vi "CRYAPI Pic Get FloatSize.vi"(7 "sAction":string, 9 "tFrameTAB":T2, 11 "tFrame":T2) -> (1 "FPPanelBound_Out":T1, 3 "tFrame_Out":T2)   [LabVIEW 2013]
uses:
  <vilib>/Utility/miscctls.llb/LVRectTypeDef.ctl
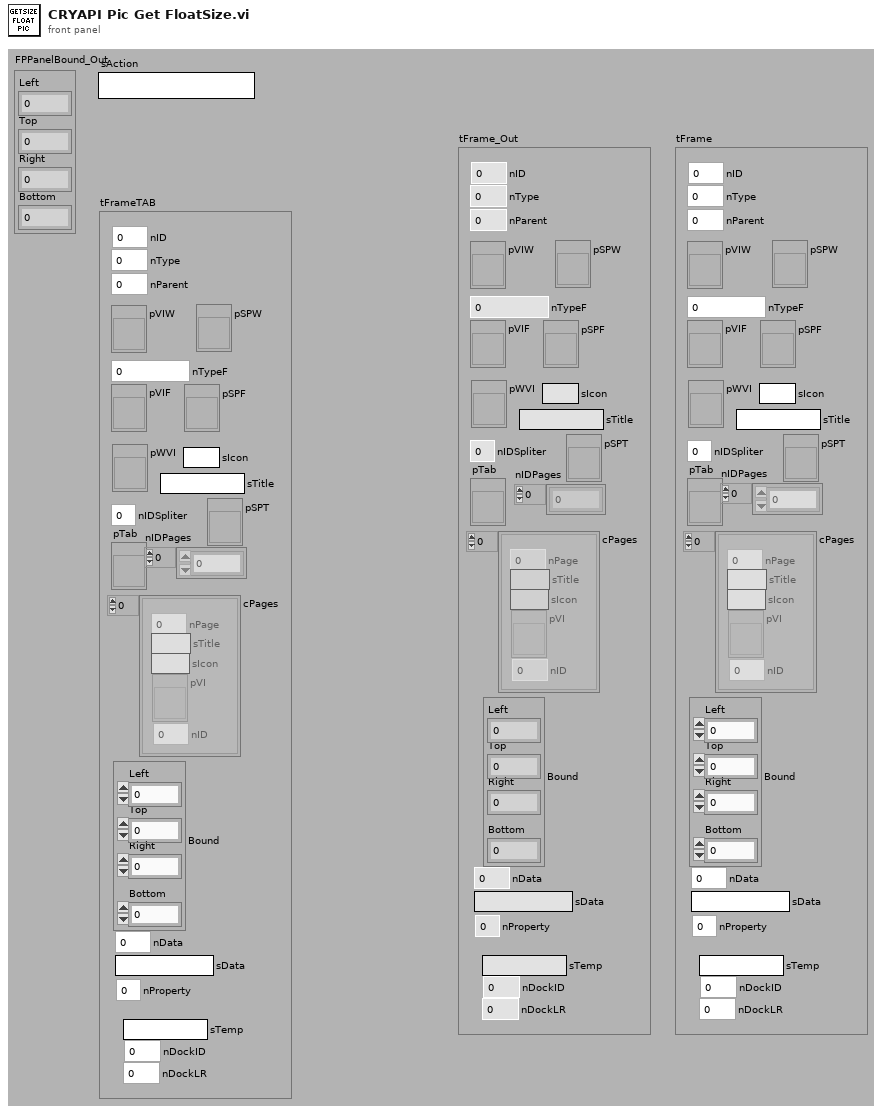
[diagram p1: front panel]
types:
  T1 = typedef "LVRectTypeDef.ctl" = cluster{"Left":i16, "Top":i16, "Right":i16, "Bottom":i16}
  T2 = cluster{"nType":i32, "nParent":i32, "pVIW":refnum<vi>, "pSPW":refnum<vi>, "nTypeF":i32, "pVIF":refnum<vi>, "pSPF":refnum<vi>, "nIDSpliter":i32, "nProperty":i32, "Bound":T1, "nID":i32, "nData":i32, "sData":string, "pWVI":refnum<vi>, "sTitle":string, "cPages":cluster{"nPage":i32, "sTitle":string, "sIcon":string, "pVI":refnum<vi>, "nID":i32}[], "pTab":refnum<vi>, "nIDPages":i32[], "pSPT":refnum<vi>, "sTemp":string, "nDockID":i32, "nDockLR":i32, "sIcon":string}
  T3 = typedef "LVBoundsTypeDef.ctl" = cluster{"Width":u32, "Height":u32}
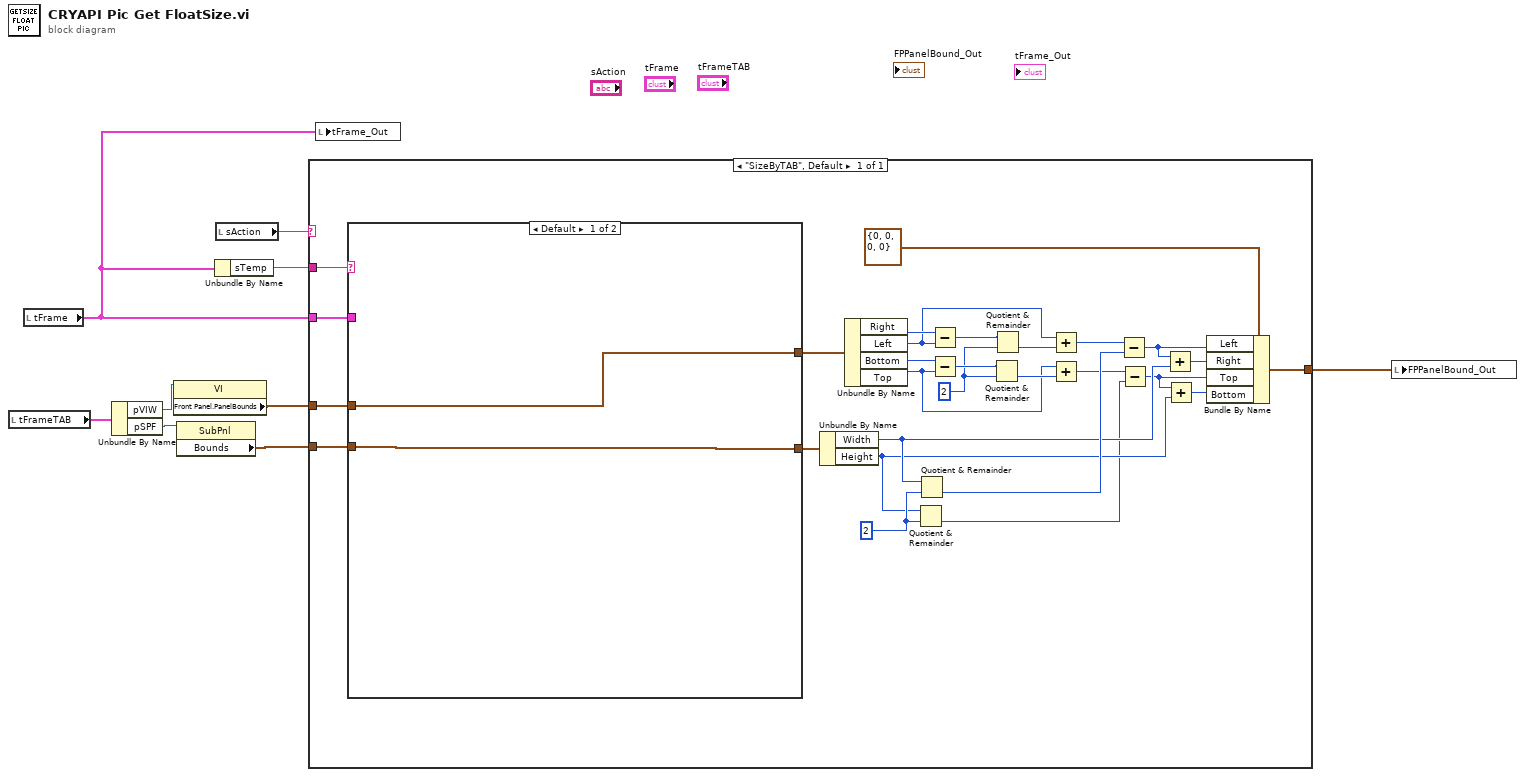
[diagram p0: block diagram]
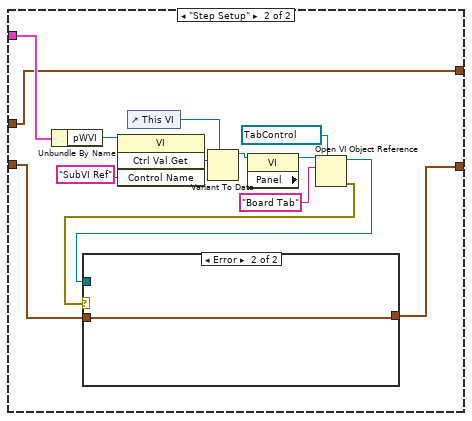
[diagram p2: hidden frame]
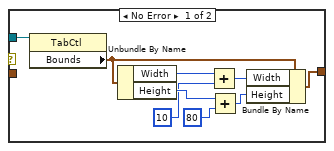
[diagram p3: hidden frame]
diagram:
  n1 = local read "tFrameTAB"() -> (w3:T2)
  n2 = local read "tFrame"() -> (w6:T2)
  n3 = Unbundle By Name(w3) -> ("pVIW"=w4:refnum<vi>, "pSPF"=w5:refnum<vi>)
  n4 = property class="VI"(reference=w4) -> ("Front Panel.PanelBounds"=w2:T1)  [unwired: 1 in, 2 out]
  n5 = property class="SubPnl"(reference=w5) -> ("Bounds"=w1:T3)  [unwired: 1 in, 2 out]
  n6 = Unbundle By Name(w6) -> ("sTemp"=w7:string)
  n7 = local read "sAction"() -> (w8:string)
  n8 = case shown="\"SizeByTAB\", Default" w8 {
    tunnel: [w14] -> w9
    tunnel: w6 -> [w12]
    tunnel: w7 -> [w13]
    tunnel: w2 -> [w11]
    tunnel: w1 -> [w10]
    frame "SizeByTAB", Default {
      w26 = 2
      w30 = 2
      n9 = case shown="Default" w13 {
        tunnel: [w39 w41] -> w37
        tunnel: [w38 w42] -> w27
        tunnel: w12 -> [_ w53]
        tunnel: w11 -> [w39 w41]
        tunnel: w10 -> [w38 w40]
        frame Default {
        }
        frame "Step Setup" {
          n10 = Unbundle By Name(w53) -> ("pWVI"=w52:refnum<vi>)
          n11 = invoke class="VI" method="Ctrl Val.Get"(reference=w52, "Control Name"="SubVI Ref") -> ("Get Control Value Variant"=w50:variant)  [unwired: 2 in, 3 out]
          n12 = control-ref of="This VI"() -> (w49:refnum<vi>)
          n13 = Variant To Data(type=w49, Variant=w50) -> (data=w47:refnum<vi>)  [unwired: 1 in, 1 out]
          n14 = property class="VI" props=["Panel"](reference=w47) -> (reference out=w46:refnum<vi>)  [unwired: 1 in, 2 out]
          n15 = Open VI Object Reference(7:refnum<vi> refnum ("Tab Control"), 10:"Board Tab" ("name/order"), 11:w46) -> (0:w44:errorcluster, 3:w43:refnum<vi>)  [unwired: 1 in]
          n16 = case shown="Error" w44 {
            tunnel: w43 -> [w62 _]
            tunnel: [w56 w63] -> w42
            tunnel: w40 -> [_ w63]
            frame No Error {
              n17 = property class="TabCtl"(reference=w62) -> ("Bounds"=w61:T3)  [unwired: 1 in, 2 out]
              n18 = Unbundle By Name(w61) -> ("Width"=w60:u32, "Height"=w59:u32)
              n19 = Add(x=w60, y=u32 10) -> (x+y=w58:u32)
              n20 = Add(x=w59, y=u32 80) -> (x+y=w57:u32)
              n21 = Bundle By Name(cluster=w61, "Width"=w58, "Height"=w57) -> (w56:T3)
            }
            frame Error {
            }
          }
        }
      }
      n22 = Unbundle By Name(w27) -> ("Width"=w22:u32, "Height"=w16:u32)
      n23 = Unbundle By Name(w37) -> ("Right"=w36:i16, "Left"=w34:i16, "Bottom"=w35:i16, "Top"=w28:i16)
      n24 = Quotient & Remainder(x=w16, y=w26) -> (floor(x/y)=w15:u32)  [unwired: 1 out]
      n25 = Quotient & Remainder(x=w22, y=w26) -> (floor(x/y)=w23:u32)  [unwired: 1 out]
      n26 = Subtract(x=w36, y=w34) -> (x-y=w33:i16)
      n27 = Subtract(x=w35, y=w28) -> (x-y=w31:i16)
      n28 = Quotient & Remainder(x=w31, y=w30) -> (floor(x/y)=w29:i32)  [unwired: 1 out]
      n29 = Quotient & Remainder(x=w33, y=w30) -> (floor(x/y)=w32:i32)  [unwired: 1 out]
      n30 = Add(x=w34, y=w32) -> (x+y=w24:i32)
      n31 = Add(x=w28, y=w29) -> (x+y=w18:i32)
      n32 = Subtract(x=w24, y=w23) -> (x-y=w21:u32)
      n33 = Subtract(x=w18, y=w15) -> (x-y=w17:u32)
      n34 = Add(x=w21, y=w22) -> (x+y=w20:u32)
      n35 = Add(x=w17, y=w16) -> (x+y=w19:u32)
      n36 = Bundle By Name(cluster=T1 {"Left"=0, "Top"=0, "Right"=0, "Bottom"=0} ("Front Panel Window:Panel Bounds"), "Left"=w21, "Right"=w20, "Top"=w17, "Bottom"=w19) -> (w14:T1)
    }
  }
  n37 = local write "tFrame_Out"(w6) -> ()
  n38 = local write "FPPanelBound_Out"(w9) -> ()
